vi "Fire User Event - Stop.vi"(8 "error in (no error)":errorcluster, 11 "userEvents":T1) -> (0 "error out":errorcluster)   [LabVIEW 2019, in "HLA Custom Device Engine.lvlib" / "User Events.lvlib"]
uses:
  User Events.lvlib
  userEvents_type.ctl
  emea-ni-adg-hla-lv/apps/generic/_typedefs/app_data.ctl
  emea-ni-adg-hla-lv/src/helpers/Dictionaries/_typedefs/object_map_type.ctl
  emea-ni-adg-hla-lv/src/helpers/Dictionaries/_typedefs/object_type.ctl
  emea-ni-adg-hla-lv/src/helpers/Dictionaries/_typedefs/attribute_map_type.ctl
  emea-ni-adg-hla-lv/src/helpers/Dictionaries/_typedefs/attribute_type.ctl
  emea-ni-adg-hla-lv/src/helpers/Dictionaries/_typedefs/lv_dataType_type.ctl
  emea-ni-adg-hla-lv/src/helpers/Dictionaries/_typedefs/interaction_map_type.ctl
  emea-ni-adg-hla-lv/src/helpers/Dictionaries/_typedefs/interaction_type.ctl
  emea-ni-adg-hla-lv/src/helpers/Dictionaries/_typedefs/parameter_map_type.ctl
  emea-ni-adg-hla-lv/src/helpers/Dictionaries/_typedefs/parameter_type.ctl
  emea-ni-adg-hla-lv/src/helpers/Dictionaries/_typedefs/instanceHandle_map_type.ctl
  objectNameNotification_type.ctl
  emea-ni-adg-hla-lv/src/helpers/ObjectManagement/ObjManager.lvlib
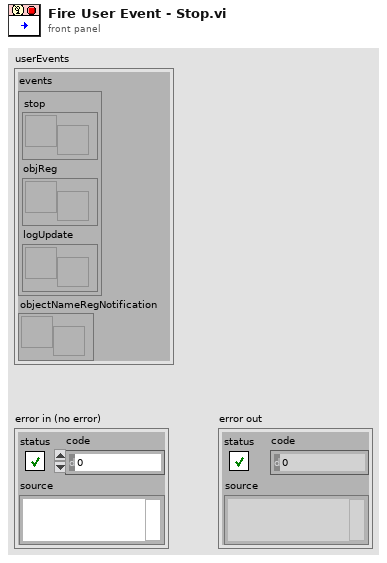
[diagram p1: front panel]
types:
  T1 = typedef "HLA Custom Device Engine.lvlib/User Events.lvlib/userEvents_type.ctl" = cluster{"events":cluster{"stop":refnum<user-event>, "objReg":refnum<user-event>, "logUpdate":refnum<user-event>}, "objectNameRegNotification":refnum<notifier>}
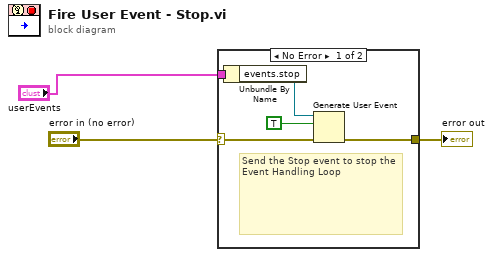
[diagram p0: block diagram]
diagram:
  n1 = case shown="No Error" "error in (no error)" {
    selector: "error in (no error)" -> [w6 w9]
    tunnel: [w7 w9] -> w3
    tunnel: "userEvents" -> [w5 _]
    frame No Error {
      # "Send the Stop event to stop the Event Handling Loop"
      n2 = Unbundle By Name(w5) -> ("events.stop"=w4:refnum<user-event>)
      n3 = Generate User Event(user event=w4, event data cluster=TRUE ("event data"), error in=w6) -> (error out=w7:errorcluster)  [unwired: 1 in, 1 out]
    }
    frame Error {
    }
  }
  "error out" <- w3
